vi "Ultrasonic_Locator.vi"() -> ()   [LabVIEW 2018]
uses:
  <vilib>/Instr/_visa.llb/VISA Configure Serial Port (Instr).vi
panel:
  in  "Clear Button":bool
  in  "stop":bool
  out "Polar Plot 2":picture
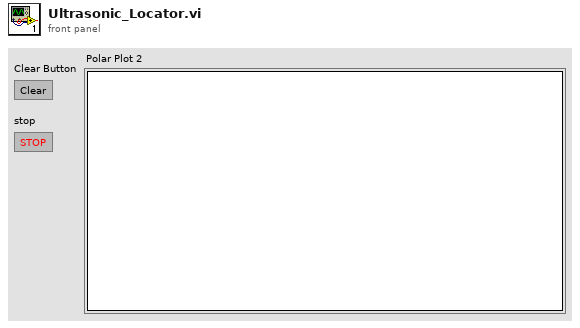
[diagram p1: front panel]
types:
  T1 = cluster{"maximum":dbl, "minimum":dbl, "clip to min":bool, "log?(F)":bool, "grid color":u32, "plot color":u32, "fmt and prec":cluster{"format":enum8{"Decimal", "Scientific", "Engineering", "Binary", "Octal", "Hex"}, "precision":u8}, "visible section":u16}
  T2 = typedef "LVBoundsTypeDef.ctl" = cluster{"Width":u32, "Height":u32}
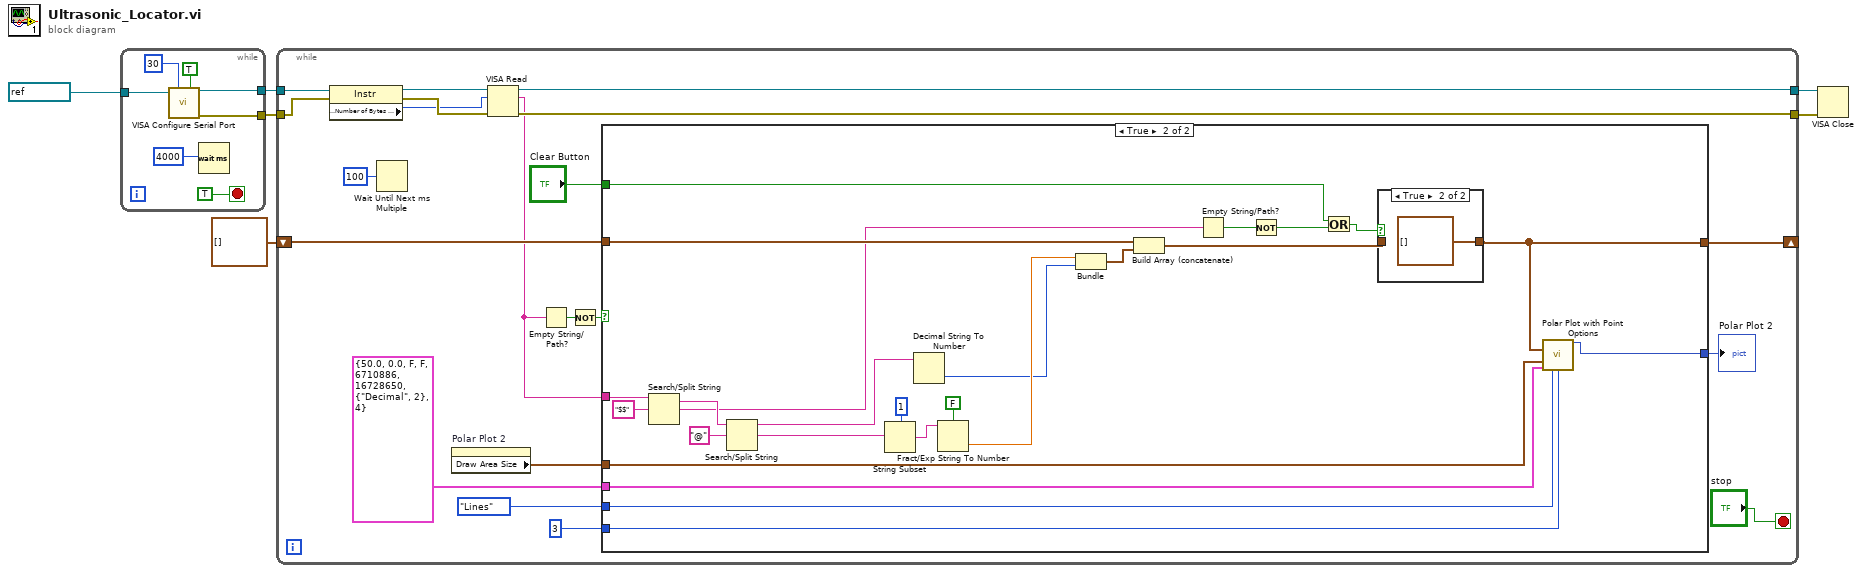
[diagram p0: block diagram]
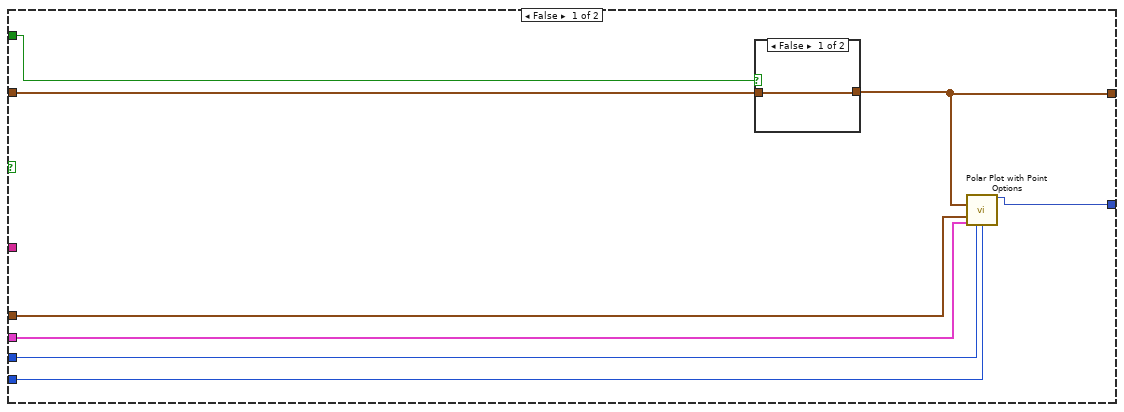
[diagram p2: hidden frame]
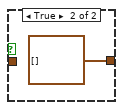
[diagram p3: hidden frame]
diagram:
  n1 = while {
    tunnel: refnum<visa-resource-name> "COM4" ("VISA resource name") -> [w10]
    tunnel: [w9] -> w3
    tunnel: [w8] -> w2
    stop <- TRUE stop-if-true
    n2 = call-poly "VISA Configure Serial Port"("VISA resource name"=w10, "timeout (10sec)"=u32 30, "Enable Termination\nChar (T)"=TRUE ("Enable Termination\nChar (T)")) -> ("VISA resource name out"=w9:refnum<visa-resource-name>, "error out"=w8:errorcluster)  [unwired: 11 in]
    n3 = Wait (ms)(milliseconds to wait=4000) -> ()  [unwired: 1 out]
  }
  n4 = while {
    tunnel: [w33] -> w5
    tunnel: [w32] -> w4
    tunnel: w3 -> [w27]
    tunnel: w2 -> [w26]
    shift-right: [w24] -> _
    shift-left: cluster{dbl, i32}[] [] -> [w25]
    stop <- "stop" stop-if-true
    n5 = property class="Instr"(reference=w27, error in=w26) -> (reference out=w31:refnum<visa-resource-name>, error out=w30:errorcluster, "Serial Settings:Number of Bytes at Serial Port"=w29:u32)
    n6 = Wait Until Next ms Multiple(millisecond multiple=u32 100 ("milliseconds to wait")) -> ()  [unwired: 1 out]
    n7 = property on="Polar Plot 2" class="Pict"() -> ("Draw Area Size"=w17:T2)  [unwired: 2 in, 2 out]
    n8 = VISA Read ("Distance")(VISA resource name=w31, byte count=w29, error in (no error)=w30) -> (VISA resource name out=w33:refnum<visa-resource-name>, read buffer=w20:string, error out=w32:errorcluster)  [unwired: 1 out]
    n9 = Empty String/Path?(string/path=w20) -> (empty?=w22:bool)
    n10 = Not(x=w22) -> (.not. x?=w21:bool)
    n11 = case shown="True" w21 {
      tunnel: w25 -> [w41 w60]
      tunnel: [w40 w59] -> w24
      tunnel: w20 -> [_ w51]
      tunnel: "Clear Button" -> [w34 w49]
      tunnel: [w39 w48] -> w18
      tunnel: w17 -> [w35 w47]
      tunnel: T1 {"maximum"=50.0, "minimum"=0.0, "clip to min"=FALSE, "log?(F)"=FALSE, "grid color"=6710886, "plot color"=16728650, "fmt and prec"={"format"=enum."Decimal", "precision"=2}, "visible section"=4} ("polar attributes") -> [w36 w46]
      tunnel: enum16{"Lines", "Points"}."Lines" ("Lines/Points") -> [w38 w44]
      tunnel: u16 3 ("Size") -> [w37 w45]
      frame False {
        n12 = case shown="False" w34 {
          tunnel: [w42 cluster{dbl, i32}[] []] -> w40
          tunnel: w41 -> [w42 _]
          frame False {
          }
          frame True {
          }
        }
        n13 = call <vilib>:"Polar Plot with Point Options.vi"("data array [mag, phase (deg)]"=w40, "dimensions (w,h)"=w35, "polar attributes"=w36, "Lines/Points"=w38, "Size"=w37) -> ("new picture"=w39:picture)  [unwired: 10 in]
      }
      frame True {
        n14 = Search/Split String(string=w51, search string/char (-)="$$") -> (substring before match=w54:string, match + rest of string=w53:string)  [unwired: 1 in, 1 out]
        n15 = Search/Split String(string=w54, search string/char (-)="@") -> (substring before match=w65:string, match + rest of string=w67:string)  [unwired: 1 in, 1 out]
        n16 = String Subset(string=w67, offset (0)=1) -> (substring=w64:string)  [unwired: 1 in]
        n17 = Decimal String To Number(string=w65) -> (number=w56:i32)  [unwired: 2 in, 1 out]
        n18 = Fract/Exp String To Number(use system decimal point (T)=FALSE, string=w64) -> (number=w63:dbl)  [unwired: 2 in, 1 out]
        n19 = Bundle(w63, w56) -> (w61:cluster{dbl, i32})  [unwired: 1 in]
        n20 = Build Array (concatenate)(w60, w61) -> (w58:cluster{dbl, i32}[])
        n21 = Empty String/Path?(string/path=w53) -> (empty?=w52:bool)
        n22 = Not(x=w52) -> (.not. x?=w50:bool)
        n23 = Or(x=w49, y=w50) -> (x .or. y?=w57:bool)
        n24 = case shown="True" w57 {
          tunnel: [w69 cluster{dbl, i32}[] []] -> w59
          tunnel: w58 -> [w69 _]
          frame False {
          }
          frame True {
          }
        }
        n25 = call <vilib>:"Polar Plot with Point Options.vi"("data array [mag, phase (deg)]"=w59, "dimensions (w,h)"=w47, "polar attributes"=w46, "Lines/Points"=w44, "Size"=w45) -> ("new picture"=w48:picture)  [unwired: 10 in]
      }
    }
    "Polar Plot 2" <- w18
  }
  n26 = VISA Close(VISA resource name=w5, error in (no error)=w4) -> ()  [unwired: 1 out]
